vi "AlazarDSPGetInfo.vi"(0 "DSP Handle":u64, 11 "error in (no error)":errorcluster) -> (1 "Module ID":u32, 2 "Version Major":u16, 3 "Version Minor":u16, 4 "DSP Handle":u64, 6 "Max Length":u32, 10 "Return Code":u32, 13 "Reserved 1":u32, 14 "Reserved 0":u32, 15 "error out":errorcluster)   [LabVIEW 2009]
uses:
  ATSApi.dll
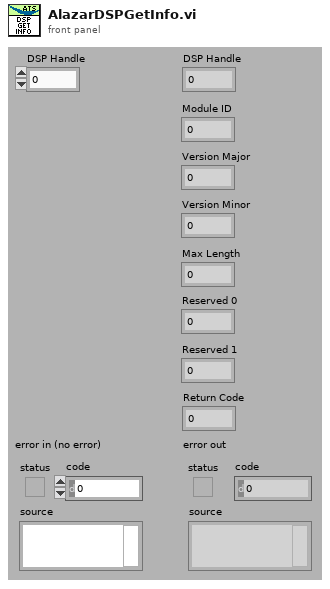
[diagram p1: front panel]
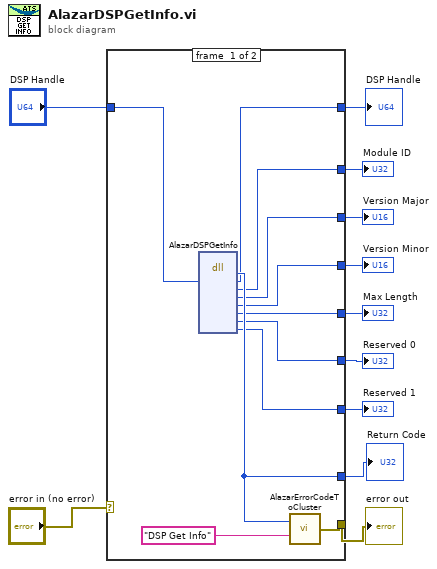
[diagram p0: block diagram]
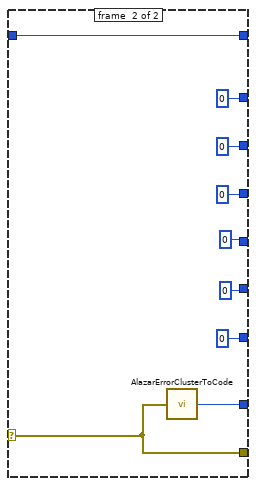
[diagram p2: hidden frame]
diagram:
  n1 = case shown="No Error" "error in (no error)" {
    selector: "error in (no error)" -> [_ w31]
    tunnel: [w19 w31] -> w10
    tunnel: [w21 w30] -> w9
    tunnel: "DSP Handle" -> [w22 w29]
    tunnel: [w18 w29] -> w7
    tunnel: [w17 0] -> w6
    tunnel: [w16 0] -> w5
    tunnel: [w15 0] -> w4
    tunnel: [w14 0] -> w3
    tunnel: [w13 0] -> w2
    tunnel: [w12 0] -> w1
    frame #0 {
      n2 = dll-call lib="ATSApi.dll" fn="AlazarDSPGetInfo"("handle"=w22) -> ("return type"=w21:u32, "handle"=w18:u64, "moduleId"=w17:u32, "versionMajor"=w16:u16, "versionMinor"=w15:u16, "maxLength"=w14:u32, "Reserved 0"=w13:u32, "Reserved 1"=w12:u32)  [unwired: 9 in, 2 out]
      n3 = call "AlazarErrorCodeToCluster.vi"("Message"="DSP Get Info", "Error Code"=w21) -> ("error out"=w19:errorcluster)
    }
    frame #1 {
      n4 = call "AlazarErrorClusterToCode.vi"("error in (no error)"=w31) -> ("Error Code"=w30:u32)
    }
  }
  "DSP Handle" <- w7
  "error out" <- w10
  "Return Code" <- w9
  "Module ID" <- w6
  "Version Major" <- w5
  "Version Minor" <- w4
  "Max Length" <- w3
  "Reserved 0" <- w2
  "Reserved 1" <- w1
